vi "TEST DRIVE.vi"() -> ()   [LabVIEW 2023]
uses:
  ctrl defs/ctrl MOTOR SELECT.ctl
  <vilib>/Rock Robotics/WPI/ThirdParty/REV Robotics/REVLib/Typedef/Spark MAX Idle Mode.ctl
  ctrl defs/ctrl swerve motor.ctl
  ctrl defs/ctrl Spark MAX current limiting.ctl
  <vilib>/Rock Robotics/WPI/MotorControl/WPI_MotorControlDeviceRef.ctl
  <vilib>/Rock Robotics/WPI/MotorControl/WPI_MotorControlType.ctl
  <vilib>/Rock Robotics/SystemInterfaces/DIO/FPGA_DIOPWMChannel.ctl
  <vilib>/Rock Robotics/WPI/PWM/WPI_PWMDeadband.ctl
  <vilib>/Rock Robotics/SystemInterfaces/DIO/FPGA_DIOChannel.ctl
  <vilib>/Rock Robotics/WPI/ThirdParty/REV Robotics/REVLib/Typedef/Spark MAX Control Type.ctl
  Global INIT.vi
panel:
  out "Sensor Velocity":dbl
  out "Sensor Position":dbl
  out "Hard Limit Rev":bool
  out "Hard Limit Fwd":bool
  in  "MOTOR %VBus":dbl(slide) scale=-1.0..1.0
  out "motors":T1[](array[typedef]) {"MOTOR SELECT" items=["REV NEO"=5676, "REV NEO 550"=11000, "VEX Falcon"=6380, "WC Kraken"=6000]}
  in  "SAFETY":bool
  in  "commit to INIT":bool
  in  "commit WRITE":bool
  in  "Idle Mode":T3
  in  "Invert":bool
  in  "refnum name":string
  in  "CAN ID":u8
  in  "Installed?":bool
  in  "MOTOR SELECT":T2 items=["REV NEO"=5676, "REV NEO 550"=11000, "VEX Falcon"=6380, "WC Kraken"=6000]
  in  "description":string
  in  "stop":bool
  in  "Select\nDRIVE motor":T5(ring)=enum."Front Left"
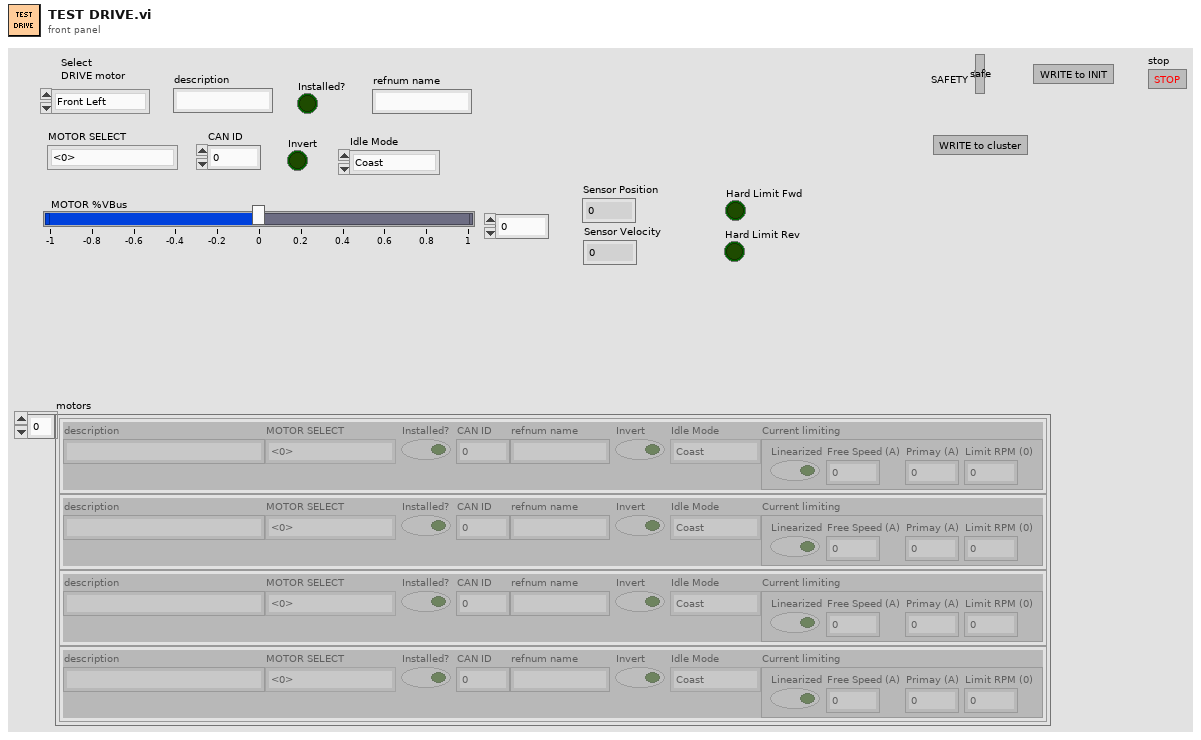
[diagram p1: front panel]
types:
  T1 = typedef "ctrl swerve motor.ctl" = cluster{"description":string, "MOTOR SELECT":T2, "Installed?":bool, "CAN ID":u8, "refnum name":string, "Invert":bool, "Idle Mode":T3, "Current limiting":T4}
  T2 = typedef "ctrl MOTOR SELECT.ctl" = i16
  T3 = typedef "Spark MAX Idle Mode.ctl" = enum16{"Coast", "Brake"}
  T4 = typedef "ctrl Spark MAX current limiting.ctl" = cluster{"Linearized":bool, "Free Speed (A)":dbl, "Primay (A)":dbl, "Limit RPM (0)":u32}
  T5 = enum16{"Front Right", "Front Left", "Rear Left", "Rear Right"}
  T6 = typedef "WPI_MotorControlDeviceRef.ctl" = cluster{"DeviceStatus":errorcluster, "Type":T7, "PWM":cluster{"PWM Channel":T8, "DeadBand":T9}, "CAN":cluster{"Device Number":u8, "SetOutput VI Ref":variant, "GetOutput VI Ref":variant, "Enable VI Ref":variant, "Disable VI Ref":variant, "Data":variant}, "Invert":bool, "DIO PWM":cluster{"PWM \"Enable\" Channel":T8, "DIOChannel":T10, "PWM Rate":dbl}}
  T7 = typedef "WPI_MotorControlType.ctl" = enum16{"PWM", "CAN", "DIO PWM"}
  T8 = typedef "FPGA_DIOPWMChannel.ctl" = enum8{"PWM 0", "PWM 1", "PWM 2", "PWM 3", "PWM 4", "PWM 5", "PWM 6", "PWM 7", "PWM 8", "PWM 9", "PWM MXP 0", "PWM MXP 1", "PWM MXP 2", "PWM MXP 3", "PWM MXP 4", "PWM MXP 5", "PWM MXP 6", "PWM MXP 7", "PWM MXP 8", "PWM MXP 9", "Invalid"}
  T9 = typedef "WPI_PWMDeadband.ctl" = cluster{"Name":string, "maxPositivePwm":i32, "minPositivePwm":i32, "centerPwm":i32, "maxNegativePwm":i32, "minNegativePwm":i32, "angularRange":u16}
  T10 = typedef "FPGA_DIOChannel.ctl" = enum8{"DIO 0", "DIO 1", "DIO 2", "DIO 3", "DIO 4", "DIO 5", "DIO 6", "DIO 7", "DIO 8", "DIO 9", "DIO MXP 0", "DIO MXP 1", "DIO MXP 2", "DIO MXP 3", "DIO MXP 4", "DIO MXP 5", "DIO MXP 6", "DIO MXP 7", "DIO MXP 8", "DIO MXP 9", "DIO MXP 10", "DIO MXP 11", "DIO MXP 12", "DIO MXP 13", "DIO MXP 14", "DIO MXP 15", "SPI Port CS1", "SPI Port CS2", "SPI Port CS3", "SPI Port MISO", "SPI Port MOSI", "Invalid"}
  T11 = typedef "Spark MAX Control Type.ctl" = enum16{"Percent VBus", "Voltage", "Velocity", "Position", "Smart Motion", "Current", "Smart Velocity"}
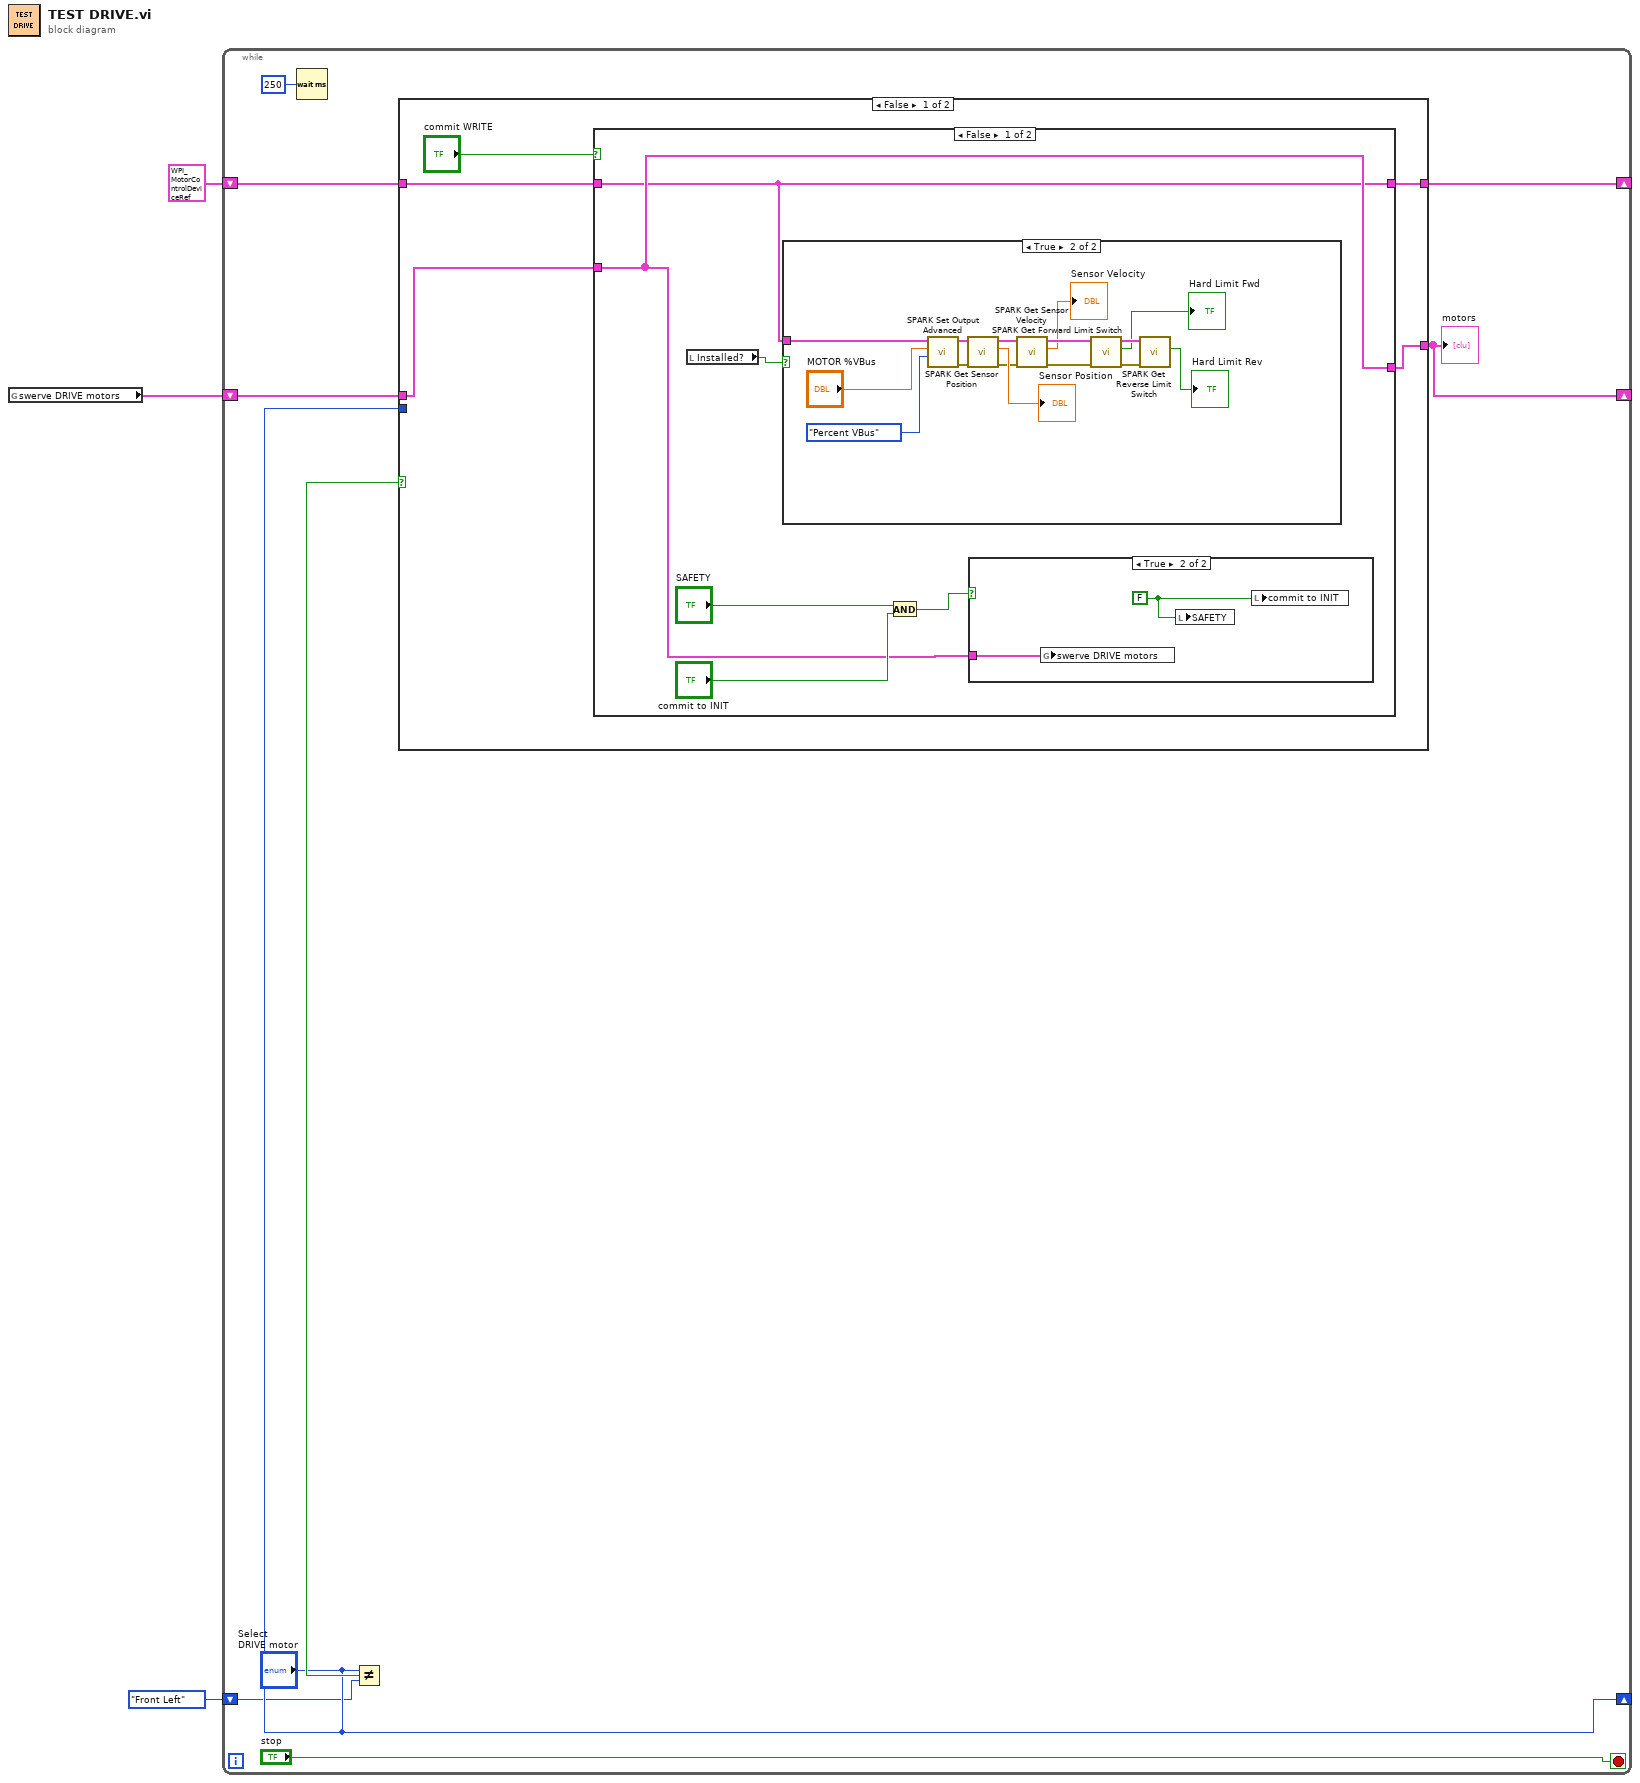
[diagram p0: block diagram]
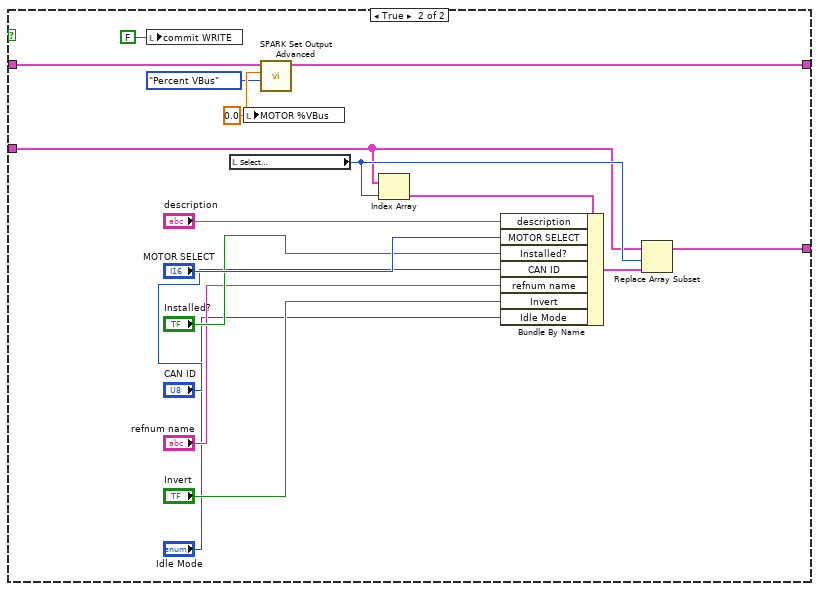
[diagram p4: hidden frame]
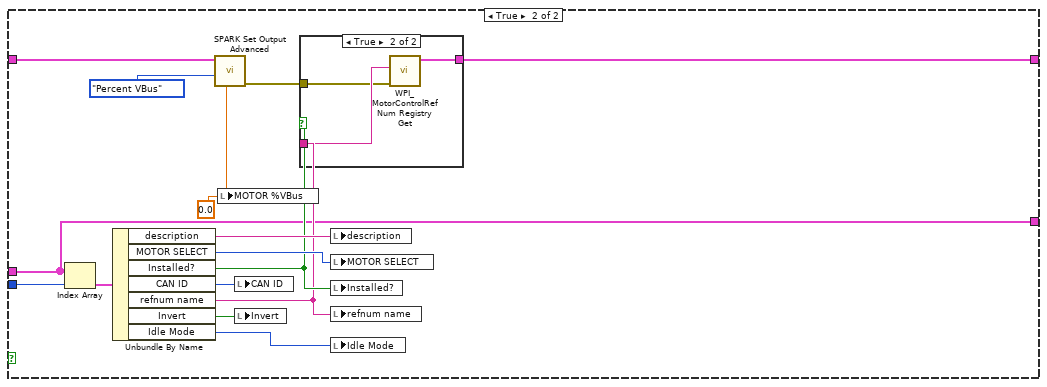
[diagram p5: hidden frame]
diagram:
  n1 = global read "Global INIT.vi" "swerve DRIVE motors"() -> (w3:T1[])
  n2 = while {
    shift-right: ["Select\nDRIVE motor"] -> _
    shift-left: T5."Front Left" ("Select\nSTEER motor") -> [w9]
    shift-right: [w7] -> _
    shift-left: w3 -> [w8]
    shift-right: [w5] -> _
    shift-left: T6 {"DeviceStatus"={"status"=FALSE, "code"=0, "source"=""}, "Type"=enum."PWM", "PWM"={"PWM Channel"=enum."Invalid", "DeadBand"={"Name"="", "maxPositivePwm"=0, "minPositivePwm"=0, "centerPwm"=0, "maxNegativePwm"=0, "minNegativePwm"=0, "angularRange"=0}}, "CAN"={"Device Number"=0, "SetOutput VI Ref"=variant, "GetOutput VI Ref"=variant, "Enable VI Ref"=variant, "Disable VI Ref"=variant, "Data"=variant}, "Invert"=FALSE, "DIO PWM"={"PWM \"Enable\" Channel"=enum."Invalid", "DIOChannel"=enum."Invalid", "PWM Rate"=0.0}} ("MotorControlDevRef") -> [w4]
    stop <- "stop" stop-if-true
    n3 = Wait (ms)(milliseconds to wait=u32 250) -> ()  [unwired: 1 out]
    n4 = Not Equal?(x="Select\nDRIVE motor", y=w9) -> (x != y?=w11:bool)
    n5 = case shown="False" w11 {
      tunnel: w8 -> [w13 w59]
      tunnel: "Select\nDRIVE motor" -> [_ w58]
      tunnel: [w16 w59] -> w7
      tunnel: [w14 w64] -> w5
      tunnel: w4 -> [w15 w61]
      frame False {
        n6 = case shown="False" "commit WRITE" {
          tunnel: w13 -> [w20 w54]
          tunnel: [w20 w56] -> w16
          tunnel: w15 -> [w18 w44]
          tunnel: [w18 w43] -> w14
          frame False {
            n7 = local read "Installed?"() -> (w19:bool)
            n8 = case shown="True" w19 {
              tunnel: w18 -> [_ w38]
              frame False {
              }
              frame True {
                n9 = call <vilib>:"SPARK Set Output Advanced.vi"("Control Mode"=Spark_MAX_Control_Type."Percent VBus", "Setpoint"="MOTOR %VBus", "MotorControlDevRef"=w38) -> ("error out"=w28:errorcluster, "MotorControlDevRef"=w29:T6)  [unwired: 7 in]
                n10 = call <vilib>:"SPARK Get Sensor Position.vi"("error in (no error)"=w28, "MotorControlDevRef in"=w29) -> ("error out"=w31:errorcluster, "Sensor Position"=→"Sensor Position":dbl, "MotorControlDevRef out"=w35:T6)  [unwired: 6 in, 1 out]
                n11 = call <vilib>:"SPARK Get Sensor Velocity.vi"("error in (no error)"=w31, "MotorControlDevRef in"=w35) -> ("error out"=w30:errorcluster, "Sensor Velocity"=→"Sensor Velocity":dbl, "MotorControlDevRef out"=w34:T6)  [unwired: 6 in, 1 out]
                n12 = call <vilib>:"SPARK Get Forward Limit Switch.vi"("error in (no error)"=w30, "MotorControlDevRef in"=w34) -> ("error out"=w24:errorcluster, "Hard Limit Fwd"=→"Hard Limit Fwd":bool, "MotorControlDevRef out"=w27:T6)  [unwired: 6 in, 1 out]
                n13 = call <vilib>:"SPARK Get Reverse Limit Switch.vi"("error in (no error)"=w24, "MotorControlDevRef in"=w27) -> ("Hard Limit Rev"=→"Hard Limit Rev":bool)  [unwired: 6 in, 3 out]
              }
            }
            n14 = And(x="SAFETY", y="commit to INIT") -> (x .and. y?=w21:bool)
            n15 = case shown="True" w21 {
              tunnel: w20 -> [_ w40]
              frame False {
              }
              frame True {
                w39 = FALSE ("SAFETY")
                n16 = global write "Global INIT.vi" "swerve DRIVE motors"(w40) -> ()
                n17 = local write "SAFETY"(w39) -> ()
                n18 = local write "commit to INIT"(w39) -> ()
              }
            }
          }
          frame True {
            w42 = 0.0 ("Setpoint")
            n19 = local write "commit WRITE"(FALSE ("commit WRITE")) -> ()
            n20 = local read "Select\nDRIVE motor"() -> (w55:T5)
            n21 = local write "MOTOR %VBus"(w42) -> ()
            n22 = call <vilib>:"SPARK Set Output Advanced.vi"("Control Mode"=Spark_MAX_Control_Type."Percent VBus", "Setpoint"=w42, "MotorControlDevRef"=w44) -> ("MotorControlDevRef"=w43:T6)  [unwired: 7 in, 1 out]
            n23 = Index Array(array=w54, index=w55) -> (element=w53:T1)
            n24 = Bundle By Name(cluster=w53, "description"="description", "MOTOR SELECT"="MOTOR SELECT", "Installed?"="Installed?", "CAN ID"="CAN ID", "refnum name"="refnum name", "Invert"="Invert", "Idle Mode"="Idle Mode") -> (w52:T1)
            n25 = Replace Array Subset(array=w54, new element=w52, index=w55) -> (w56:T1[])
          }
        }
      }
      frame True {
        w63 = 0.0 ("Setpoint")
        n26 = Index Array(array=w59, index=w58) -> (element=w72:T1)
        n27 = Unbundle By Name(w72) -> ("description"=w71:string, "MOTOR SELECT"=w69:T2, "Installed?"=w66:bool, "CAN ID"=w67:u8, "refnum name"=w65:string, "Invert"=w68:bool, "Idle Mode"=w70:T3)
        n28 = call <vilib>:"SPARK Set Output Advanced.vi"("Control Mode"=Spark_MAX_Control_Type."Percent VBus", "Setpoint"=w63, "MotorControlDevRef"=w61) -> ("error out"=w60:errorcluster)  [unwired: 7 in, 1 out]
        n29 = local write "MOTOR %VBus"(w63) -> ()
        n30 = local write "CAN ID"(w67) -> ()
        n31 = local write "Invert"(w68) -> ()
        n32 = case shown="True" w66 {
          tunnel: w65 -> [_ w75]
          tunnel: [_ w74] -> w64
          tunnel: w60 -> [_ w73]
          frame False {
          }
          frame True {
            n33 = call <vilib>:"WPI_MotorControlRefNum Registry Get.vi"("error in (no error)"=w73, "refnum name"=w75) -> ("MotorControlDevRef"=w74:T6)  [unwired: 8 in, 1 out]
          }
        }
        n34 = local write "description"(w71) -> ()
        n35 = local write "MOTOR SELECT"(w69) -> ()
        n36 = local write "Installed?"(w66) -> ()
        n37 = local write "refnum name"(w65) -> ()
        n38 = local write "Idle Mode"(w70) -> ()
      }
    }
    "motors" <- w7
  }
